vi "Test.vi"() -> ()   [LabVIEW 2014]
doc: "This VI is called when test mode begins, and will automatically be terminated when it ends. You can add manual or automatic tests and invoke them from the dashboard."
panel:
  out "Power level":dbl(graph)
  out "Index":i32
  out "Power Level":dbl
  out "Motor Speed":cluster{"Rate":dbl}(graph)
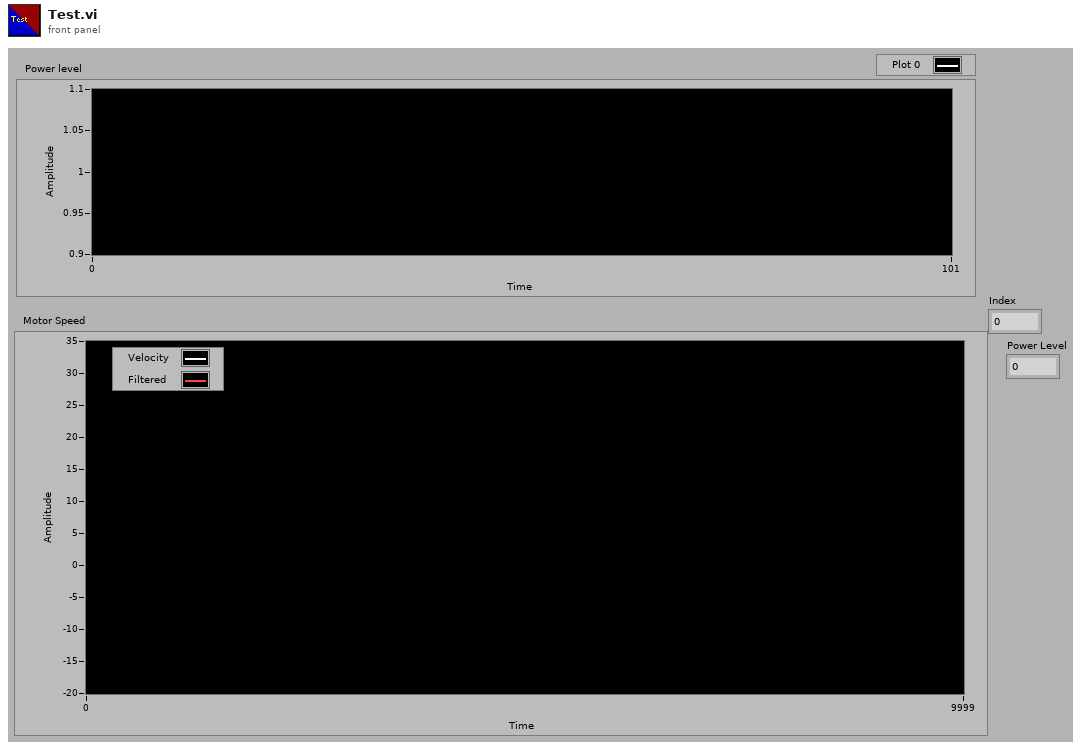
[diagram p1: front panel]
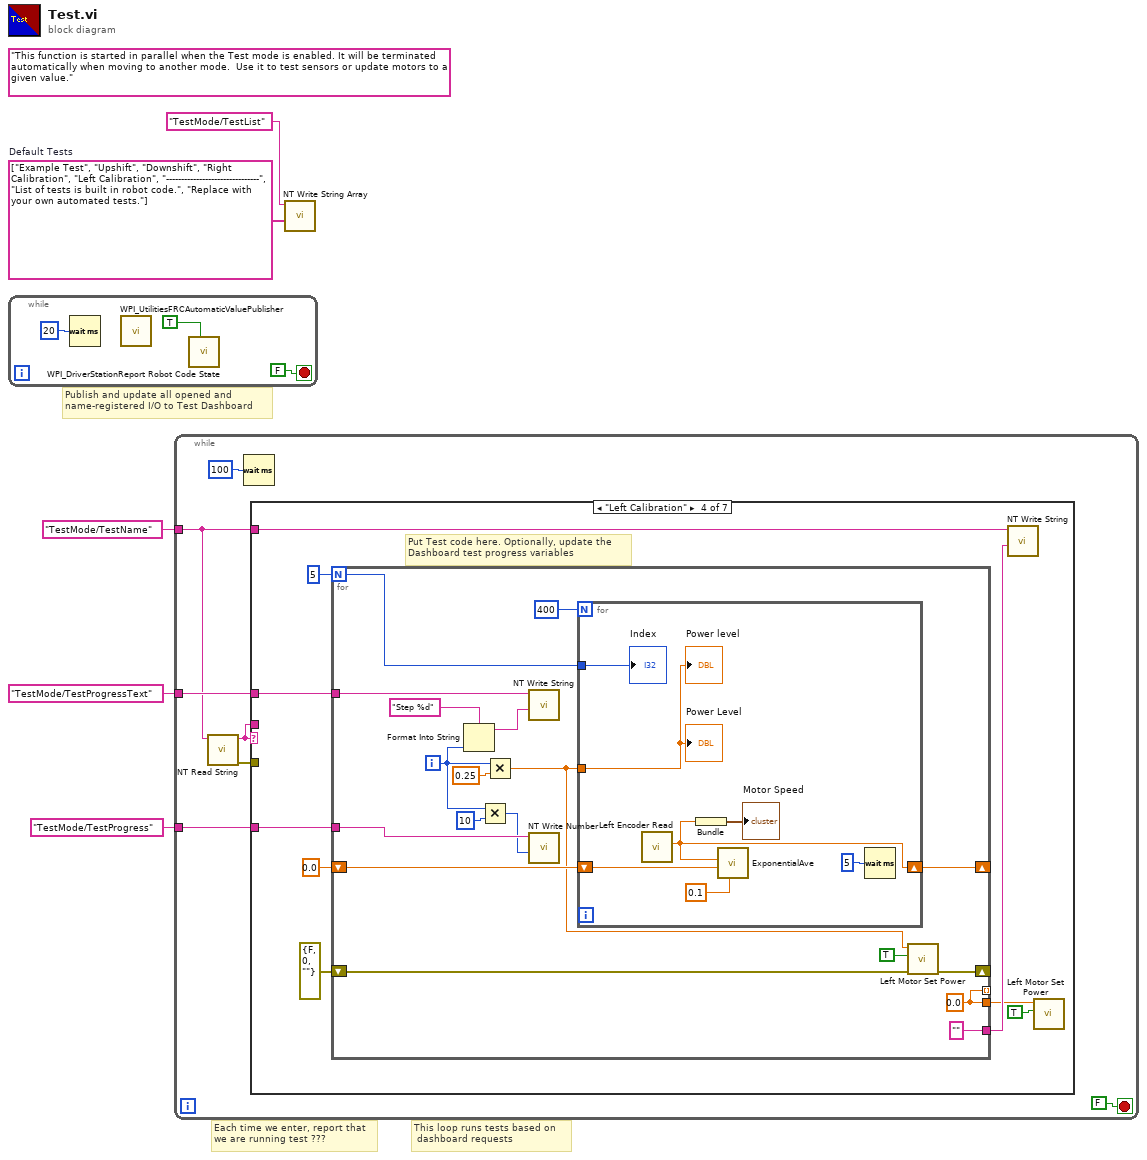
[diagram p0: block diagram]
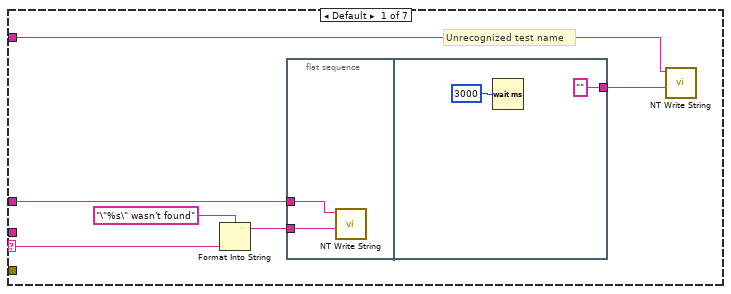
[diagram p2: hidden frame]
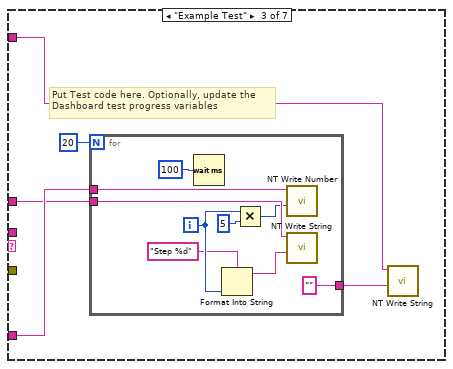
[diagram p4: hidden frame]
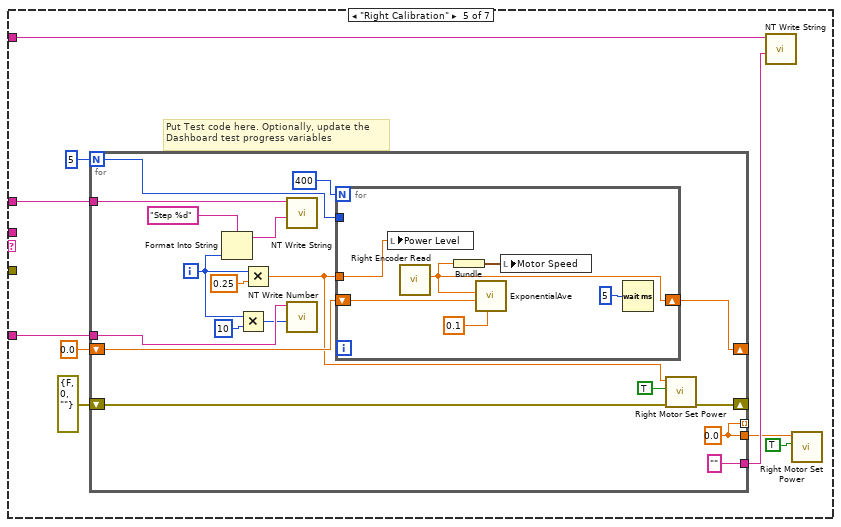
[diagram p5: hidden frame]
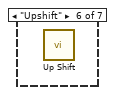
[diagram p6: hidden frame]
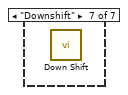
[diagram p7: hidden frame]
diagram:
  w2 = string[] ["Example Test", "Upshift", "Downshift", "Right Calibration", "Left Calibration", "-------------------------------", "List of tests is built in robot code.", "Replace with your own automated tests."]  # Default Tests
  (unwired) "This function is started in parallel when the Test mode is enabled. It will be terminated automatically when moving to another mode.  Use it to test sensors or update motors to a given value."
  # "This loop runs tests based on \n dashboard requests"
  # "Publish and update all opened and\nname-registered I/O to Test Dashboard"
  # "Each time we enter, report that\nwe are running test ???"
  n1 = while {
    stop <- FALSE stop-if-true
    n2 = Wait (ms)(milliseconds to wait=u32 20) -> ()  [unwired: 1 out]
    n3 = call <vilib>:"WPI_UtilitiesFRCAutomaticValuePublisher.vi"() -> ()  [unwired: 12 in]
    n4 = call <vilib>:"WPI_DriverStationReport Robot Code State.vi"("Test"=TRUE ("Autonomous")) -> ()  [unwired: 10 in, 1 out]
  }
  n5 = while {
    tunnel: "TestMode/TestName" ("Name") -> [w10]
    tunnel: "TestMode/TestProgressText" ("Name") -> [w13]
    tunnel: "TestMode/TestProgress" ("Name") -> [w12]
    stop <- FALSE stop-if-true
    n6 = call <vilib>:"NT Read String.vi"("Name"=w10) -> ("error out"=w9:errorcluster, "String"=w11:string)  [unwired: 9 in]
    n7 = Wait (ms)(milliseconds to wait=u32 100) -> ()  [unwired: 1 out]
    n8 = case shown="\"Left Calibration\"" w11 {
      selector: w11 -> [w20 _ _ _ _ _ _]
      tunnel: w10 -> [w17 _ w26 w44 w78 _ _]
      tunnel: w13 -> [w21 _ w29 w47 w81 _ _]
      tunnel: w12 -> [_ _ w30 w48 w82 _ _]
      tunnel: w11 -> [_ _ _ _ _ _ _]
      tunnel: w9 -> [_ _ _ _ _ _ _]
      frame Default {
        # "Unrecognized test name"
        n9 = Format Into String(format string="\"%s\" wasn't found" ("Name"), w20) -> (resulting string=w19:string)  [unwired: 2 in, 1 out]
        n10 = flat-sequence {
          tunnel: w21 -> [w22]
          tunnel: w19 -> [w23]
          tunnel: ["" ("Name")] -> w16
          frame #0 {
            n11 = call <vilib>:"NT Write String.vi"("String"=w23, "Name"=w22) -> ()  [unwired: 9 in, 1 out]
          }
          frame #1 {
            n12 = Wait (ms)(milliseconds to wait=u32 3000) -> ()  [unwired: 1 out]
          }
        }
        n13 = call <vilib>:"NT Write String.vi"("String"=w16, "Name"=w17) -> ()  [unwired: 9 in, 1 out]
      }
      frame "" {
        # "No test to run"
      }
      frame "Example Test" {
        # "Put Test code here. Optionally, update the\nDashboard test progress variables"
        n14 = for {
          N: 20 -> [_]
          tunnel: w30 -> [w39]
          tunnel: w29 -> [w37]
          tunnel: ["" ("String")] -> w27
          i -> [w34]
          n15 = Wait (ms)(milliseconds to wait=u32 100) -> ()  [unwired: 1 out]
          n16 = Format Into String(format string="Step %d", w34) -> (resulting string=w32:string)  [unwired: 2 in, 1 out]
          n17 = Multiply(x=w34, y=u32 5 ("milliseconds to wait")) -> (x*y=w35:u32)
          n18 = call <vilib>:"NT Write Number.vi"("Numeric"=w35, "Name"=w39) -> ()  [unwired: 9 in, 1 out]
          n19 = call <vilib>:"NT Write String.vi"("String"=w32, "Name"=w37) -> ()  [unwired: 9 in, 1 out]
        }
        n20 = call <vilib>:"NT Write String.vi"("String"=w27, "Name"=w26) -> ()  [unwired: 9 in, 1 out]
      }
      frame "Left Calibration" {
        # "Put Test code here. Optionally, update the\nDashboard test progress variables"
        n21 = for {
          N: 5 -> [w51]
          tunnel: w48 -> [w66]
          tunnel: w47 -> [w65]
          tunnel: ["" ("String")] -> w45
          tunnel: [w59] -> w43
          tunnel: [w59] -> _ mode=indexing
          shift-right: [w55] -> _
          shift-left: 0.0 -> [w56]
          shift-right: [w53] -> _
          shift-left: errorcluster {"status"=FALSE, "code"=0, "source"=""} ("error in") -> [w54]
          i -> [w49]
          w59 = 0.0
          n22 = Format Into String(format string="Step %d", w49) -> (resulting string=w61:string)  [unwired: 2 in, 1 out]
          n23 = Multiply(x=w49, y=u32 10 ("milliseconds to wait")) -> (x*y=w63:u32)
          n24 = Multiply(x=w49, y=0.25) -> (x*y=w52:dbl)
          n25 = call <vilib>:"NT Write String.vi"("String"=w61, "Name"=w65) -> ()  [unwired: 9 in, 1 out]
          n26 = call <vilib>:"NT Write Number.vi"("Numeric"=w63, "Name"=w66) -> ()  [unwired: 9 in, 1 out]
          n27 = for {
            N: 400 -> [_]
            shift-right: [w71] -> w55
            shift-left: w56 -> [w70]
            tunnel: w52 -> [w67]
            tunnel: w51 -> [w68]
            n28 = call "Left Encoder Read.vi"() -> ("Rate"=w71:dbl)  [unwired: 8 in, 3 out]
            n29 = Bundle("Rate"=w71) -> (→"Motor Speed":cluster{"Rate":dbl})  [unwired: 1 in]
            n30 = call "ExponentialAve.vi"("Coff"=0.1, "PreviousValue"=w70, "InputValue"=w71) -> ()  [unwired: 8 in, 1 out]
            n31 = Wait (ms)(milliseconds to wait=u32 5) -> ()  [unwired: 1 out]
            "Power Level" <- w67
            "Index" <- w68
            "Power level" <- w67
          }
          n32 = call "Left Motor Set Power.vi"("error in"=w54, "Disable Ramp"=TRUE, "Output"=w52) -> ("error out"=w53:errorcluster)  [unwired: 8 in]
        }
        n33 = call <vilib>:"NT Write String.vi"("String"=w45, "Name"=w44) -> ()  [unwired: 9 in, 1 out]
        n34 = call "Left Motor Set Power.vi"("Disable Ramp"=TRUE, "Output"=w43) -> ()  [unwired: 9 in, 1 out]
      }
      frame "Right Calibration" {
        # "Put Test code here. Optionally, update the\nDashboard test progress variables"
        n35 = for {
          N: 5 -> [w85]
          tunnel: w82 -> [w100]
          tunnel: w81 -> [w99]
          tunnel: ["" ("String")] -> w79
          tunnel: [w93] -> w77
          tunnel: [w93] -> _ mode=indexing
          shift-right: [w89] -> _
          shift-left: 0.0 -> [w90]
          shift-right: [w87] -> _
          shift-left: errorcluster {"status"=FALSE, "code"=0, "source"=""} ("error in") -> [w88]
          i -> [w83]
          w93 = 0.0
          n36 = Format Into String(format string="Step %d", w83) -> (resulting string=w95:string)  [unwired: 2 in, 1 out]
          n37 = Multiply(x=w83, y=u32 10 ("milliseconds to wait")) -> (x*y=w97:u32)
          n38 = Multiply(x=w83, y=0.25) -> (x*y=w86:dbl)
          n39 = call <vilib>:"NT Write String.vi"("String"=w95, "Name"=w99) -> ()  [unwired: 9 in, 1 out]
          n40 = call <vilib>:"NT Write Number.vi"("Numeric"=w97, "Name"=w100) -> ()  [unwired: 9 in, 1 out]
          n41 = for {
            N: 400 -> [_]
            shift-right: [w105] -> w89
            shift-left: w90 -> [w104]
            tunnel: w86 -> [w101]
            tunnel: w85 -> [_]
            n42 = local write "Power Level"(w101) -> ()
            n43 = call "Right Encoder Read.vi"() -> ("Rate"=w105:dbl)  [unwired: 8 in, 3 out]
            n44 = Bundle("Rate"=w105) -> (w102:cluster{"Rate":dbl})  [unwired: 1 in]
            n45 = call "ExponentialAve.vi"("Coff"=0.1, "PreviousValue"=w104, "InputValue"=w105) -> ()  [unwired: 8 in, 1 out]
            n46 = local write "Motor Speed"(w102) -> ()
            n47 = Wait (ms)(milliseconds to wait=u32 5) -> ()  [unwired: 1 out]
          }
          n48 = call "Right Motor Set Power.vi"("error in"=w88, "Disable Ramp"=TRUE, "Output"=w86) -> ("error out"=w87:errorcluster)  [unwired: 8 in]
        }
        n49 = call <vilib>:"NT Write String.vi"("String"=w79, "Name"=w78) -> ()  [unwired: 9 in, 1 out]
        n50 = call "Right Motor Set Power.vi"("Disable Ramp"=TRUE, "Output"=w77) -> ()  [unwired: 9 in, 1 out]
      }
      frame "Upshift" {
        n51 = call "Up Shift.vi"() -> ()  [unwired: 11 in, 1 out]
      }
      frame "Downshift" {
        n52 = call "Down Shift.vi"() -> ()  [unwired: 11 in, 1 out]
      }
    }
  }
  n53 = call <vilib>:"NT Write String Array.vi"("String Array"=w2, "Name"="TestMode/TestList") -> ()  [unwired: 9 in, 1 out]
